vi "Autonomous.vi"   [LabVIEW 2017]
doc: "This VI starts when autonomous period begins, and will automatically be terminated when it ends. You can carry out timed or sensor driven operations directly to I/O or to subsystems without needing to return to the caller."
uses:
  Framework/Robot Global Data.vi
  <vilib>/Rock Robotics/Network Tables/NT Read String.vi
types:
  T1 = enum16{"Robot Position from the FMS", "Robot Position from the Dashboard", "Robot Position for Debug"}
  T2 = typedef "WPI_DriverStationPositionInfo.ctl" = enum16{"1", "2", "3"}
  T3 = cluster{"Auto Option":string, "Left Setpoint":dbl, "Right Setpoint":dbl, "Duration":dbl}[]
  T4 = typedef "Command Status Info.ctl" = cluster{"Name":string, "Status":T5, "notifier out":T6}
  T5 = typedef "Completion Status.ctl" = enum16{"Successful", "Aborted", "Incomplete"}
  T6 = typedef "Completion Notifier.ctl" = refnum<notifier>
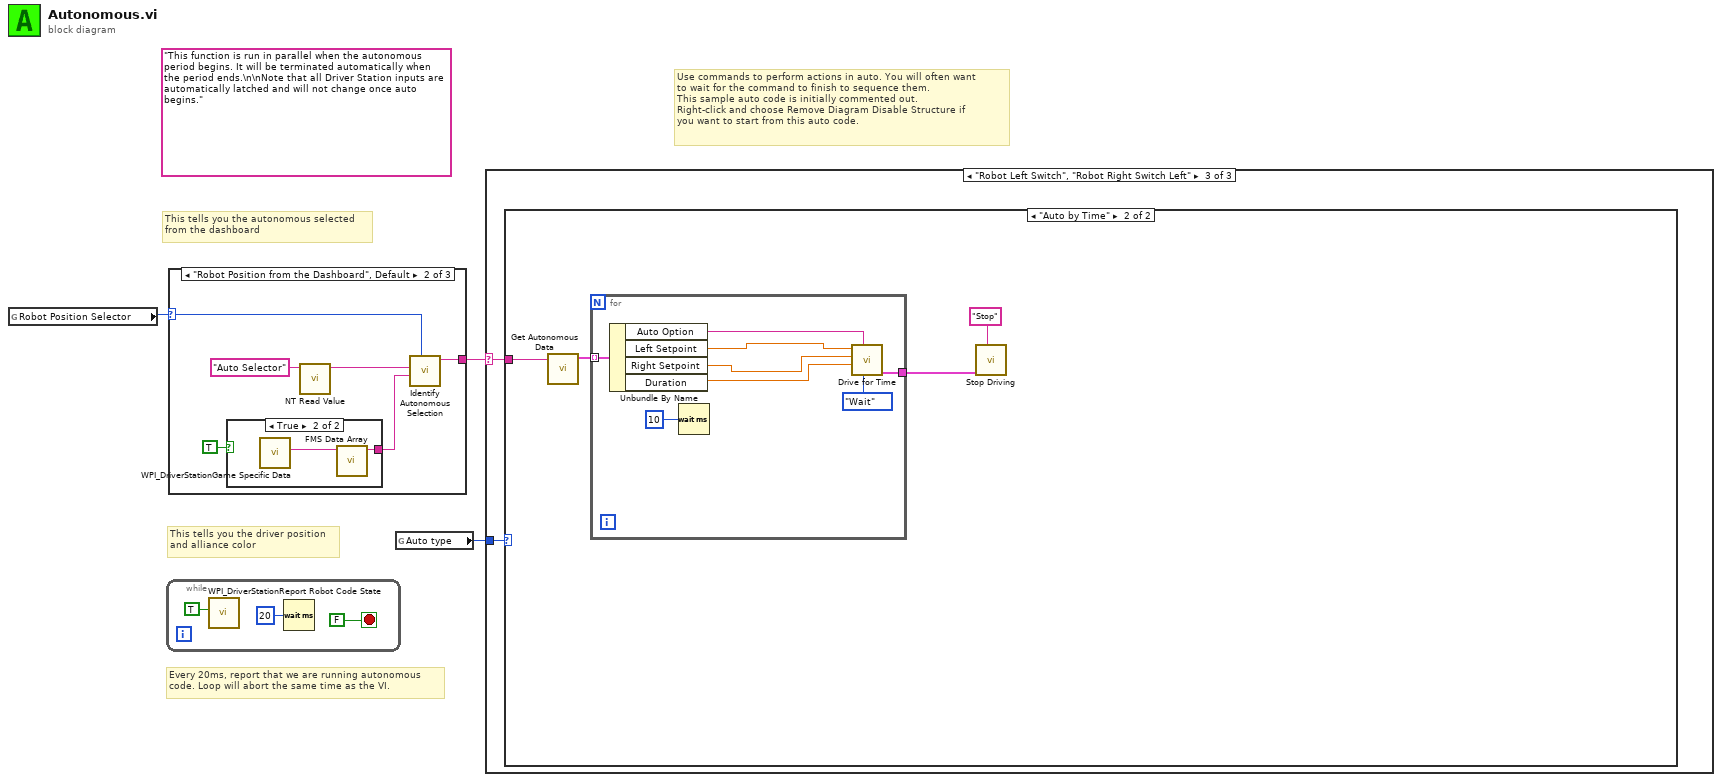
[diagram p0: block diagram]
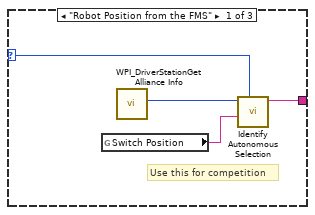
[diagram p2: hidden frame]
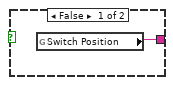
[diagram p3: hidden frame]
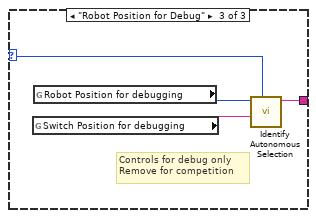
[diagram p4: hidden frame]
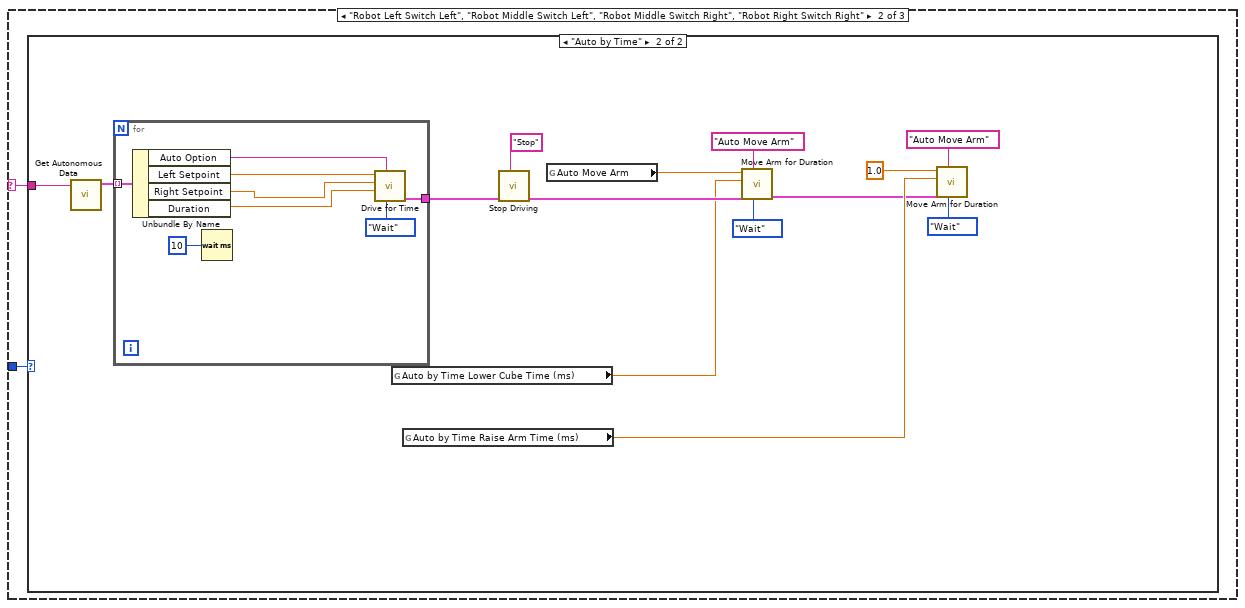
[diagram p6: hidden frame]
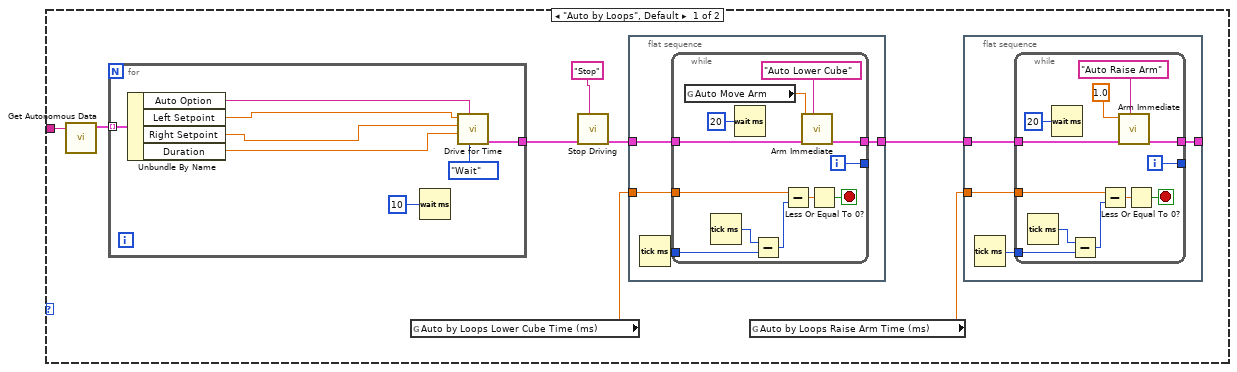
[diagram p7: hidden frame]
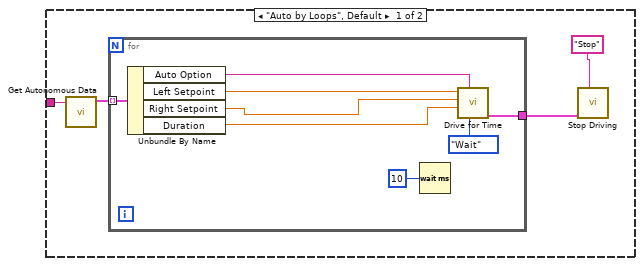
[diagram p8: hidden frame]
diagram:
  (unwired) "This function is run in parallel when the autonomous period begins. It will be terminated automatically when the period ends.\n\nNote that all Driver Station inputs are automatically latched and will not change once auto begins."
  # "This tells you the autonomous selected\nfrom the dashboard"
  # "Every 20ms, report that we are running autonomous\ncode. Loop will abort the same time as the VI."
  # "Use commands to perform actions in auto. You will often want\nto wait for the command to finish to sequence them.\nThis sample auto code is initially commented out. \nRight-click and choose Remove Diagram Disable Structure if\nyou want to start from this auto code."
  # "This tells you the driver position\nand alliance color"
  n1 = global read "Robot Global Data.vi" "Robot Position Selector"() -> (w1:T1)
  n2 = while {
    stop <- FALSE stop-if-true
    n3 = call <vilib>:"WPI_DriverStationReport Robot Code State.vi"("Autonomous"=TRUE) -> ()  [unwired: 10 in, 1 out]
    n4 = Wait (ms)(milliseconds to wait=u32 20) -> ()  [unwired: 1 out]
  }
  n5 = case shown="\"Robot Position from the Dashboard\", Default" w1 {
    selector: w1 -> [w7 w13 w20]
    tunnel: [w8 w14 w23] -> w3
    frame "Robot Position from the FMS" {
      # "Use this for competition"
      n6 = global read "Robot Global Data.vi" "Switch Position"() -> (w10:string)
      n7 = call <vilib>:"WPI_DriverStationGet Alliance Info.vi"() -> ("Position"=w9:T2)  [unwired: 11 out]
      n8 = call "Identify Autonomous Selection.vi"("Robot Position Selector"=w7, "Switch Position"=w10, "Robot Position"=w9) -> ("Autonomous Selection"=w8:string)  [unwired: 8 in]
    }
    frame "Robot Position from the Dashboard", Default {
      n9 = case shown="True" TRUE {
        tunnel: [w17 w18] -> w12
        frame False {
          n10 = global read "Robot Global Data.vi" "Switch Position"() -> (w17:string)
        }
        frame True {
          n11 = call <vilib>:"WPI_DriverStationGame Specific Data.vi"() -> ("Game Specific Data"=w19:string)  [unwired: 11 in]
          n12 = call "FMS Data Array.vi"("Game Data"=w19) -> ("Switch"=w18:string)  [unwired: 8 in, 2 out]
        }
      }
      n13 = call-poly <vilib>:"NT Read Value.vi"("Name"="Auto Selector") -> ("String"=w16:string)  [unwired: 9 in, 1 out]
      n14 = call "Identify Autonomous Selection.vi"("Robot Position Selector"=w13, "Switch Position"=w12, "Robot Position From Dashboard"=w16) -> ("Autonomous Selection"=w14:string)  [unwired: 8 in]
    }
    frame "Robot Position for Debug" {
      # "Controls for debug only\nRemove for competition"
      n15 = global read "Robot Global Data.vi" "Switch Position for debugging"() -> (w21:string)
      n16 = global read "Robot Global Data.vi" "Robot Position for debugging"() -> (w22:T2)
      n17 = call "Identify Autonomous Selection.vi"("Robot Position Selector"=w20, "Switch Position"=w21, "Robot Position"=w22) -> ("Autonomous Selection"=w23:string)  [unwired: 8 in]
    }
  }
  n18 = global read "Robot Global Data.vi" "Auto type"() -> (w2:enum16{"Auto by Time", "Auto by Loops"})
  n19 = case shown="\"Robot Left Switch\", \"Robot Right Switch Left\"" w3 {
    selector: w3 -> [_ w25 w97]
    tunnel: w2 -> [_ w24 w96]
    frame Default {
      # "You can put your main auto here, or you can right-click on the case and make any\nother frame be the default case."
      # "This is the frame that will execute if no selection is made, or if it is not recognized"
    }
    frame "Robot Left Switch Left", "Robot Middle Switch Left", "Robot Middle Switch Right", "Robot Right Switch Right" {
      n20 = case shown="\"Auto by Time\"" w24 {
        tunnel: w25 -> [w33 w87]
        frame "Auto by Loops", Default {
          n21 = call "Get Autonomous Data.vi"("Autonomous Selectin"=w33) -> ("Autonomous Data Selected"=w32:T3)  [unwired: 10 in]
          n22 = for {
            tunnel: w32 -> [w39] mode=indexing
            tunnel: [w37] -> w30
            n23 = Unbundle By Name(w39) -> ("Auto Option"=w38:string, "Left Setpoint"=w34:dbl, "Right Setpoint"=w35:dbl, "Duration"=w36:dbl)
            n24 = Wait (ms)(milliseconds to wait=u32 10 ("millisecond timer value")) -> ()  [unwired: 1 out]
            n25 = call "Drive for Time.vi"("Synchronization"=enum16{"Start", "Wait"}."Wait" ("Synchronication"), "Description"=w38, "Duration (ms)"=w36, "Right Speed"=w35, "Left Speed"=w34) -> ("Command Info Out"=w37:T4)  [unwired: 5 in, 1 out]
          }
          n26 = global read "Robot Global Data.vi" "Auto by Loops Lower Cube Time (ms)"() -> (w28:dbl)
          n27 = call "Stop Driving.vi"("Description"="Stop", "Command Info In"=w30) -> ("Command Info Out"=w29:T4)  [unwired: 9 in]
          n28 = flat-sequence {
            tunnel: [w60] -> w26
            tunnel: w29 -> [w59]
            tunnel: w28 -> [w58]
            frame #0 {
              n29 = Tick Count (ms)() -> (millisecond timer value=w61:u32)
              n30 = while {
                tunnel: w61 -> [w70]
                tunnel: w59 -> [w66]
                tunnel: [w65] -> w60
                tunnel: [w67] -> _
                tunnel: w58 -> [w63]
                i -> [w67]
                stop <- w71 stop-if-true
                n31 = global read "Robot Global Data.vi" "Auto Move Arm"() -> (w62:dbl)
                n32 = Tick Count (ms)() -> (millisecond timer value=w69:u32)
                n33 = Wait (ms)(milliseconds to wait=u32 20) -> ()  [unwired: 1 out]
                n34 = Subtract(x=w69, y=w70) -> (x-y=w73:u32)
                n35 = Subtract(x=w63, y=w73) -> (x-y=w72:dbl)
                n36 = call "Arm Immediate.vi"("Description"="Auto Lower Cube", "Command Info In"=w66, "Setpoint"=w62) -> ("Command Info Out"=w65:T4)  [unwired: 8 in]
                n37 = Less Or Equal To 0?(x=w72) -> (x <= 0?=w71:bool)
              }
            }
          }
          n38 = global read "Robot Global Data.vi" "Auto by Loops Raise Arm Time (ms)"() -> (w27:dbl)
          n39 = flat-sequence {
            tunnel: [w44] -> _
            tunnel: w26 -> [w43]
            tunnel: w27 -> [w42]
            frame #0 {
              n40 = Tick Count (ms)() -> (millisecond timer value=w45:u32)
              n41 = while {
                tunnel: w45 -> [w54]
                tunnel: w43 -> [w50]
                tunnel: [w49] -> w44
                tunnel: [w51] -> _
                tunnel: w42 -> [w46]
                i -> [w51]
                stop <- w55 stop-if-true
                n42 = Tick Count (ms)() -> (millisecond timer value=w53:u32)
                n43 = Wait (ms)(milliseconds to wait=u32 20) -> ()  [unwired: 1 out]
                n44 = Subtract(x=w53, y=w54) -> (x-y=w57:u32)
                n45 = Subtract(x=w46, y=w57) -> (x-y=w56:dbl)
                n46 = call "Arm Immediate.vi"("Description"="Auto Raise Arm", "Command Info In"=w50, "Setpoint"=1.0) -> ("Command Info Out"=w49:T4)  [unwired: 8 in]
                n47 = Less Or Equal To 0?(x=w56) -> (x <= 0?=w55:bool)
              }
            }
          }
        }
        frame "Auto by Time" {
          n48 = call "Get Autonomous Data.vi"("Autonomous Selectin"=w87) -> ("Autonomous Data Selected"=w86:T3)  [unwired: 10 in]
          n49 = for {
            tunnel: w86 -> [w93] mode=indexing
            tunnel: [w91] -> w84
            n50 = Unbundle By Name(w93) -> ("Auto Option"=w92:string, "Left Setpoint"=w88:dbl, "Right Setpoint"=w89:dbl, "Duration"=w90:dbl)
            n51 = Wait (ms)(milliseconds to wait=u32 10 ("millisecond timer value")) -> ()  [unwired: 1 out]
            n52 = call "Drive for Time.vi"("Synchronization"=enum16{"Start", "Wait"}."Wait" ("Synchronication"), "Description"=w92, "Duration (ms)"=w90, "Right Speed"=w89, "Left Speed"=w88) -> ("Command Info Out"=w91:T4)  [unwired: 5 in, 1 out]
          }
          n53 = global read "Robot Global Data.vi" "Auto by Time Lower Cube Time (ms)"() -> (w77:dbl)
          n54 = global read "Robot Global Data.vi" "Auto by Time Raise Arm Time (ms)"() -> (w76:dbl)
          n55 = call "Stop Driving.vi"("Description"="Stop", "Command Info In"=w84) -> ("Command Info Out"=w83:T4)  [unwired: 9 in]
          n56 = global read "Robot Global Data.vi" "Auto Move Arm"() -> (w74:dbl)
          n57 = call "Move Arm for Duration.vi"("Synchronization"=enum16{"Start", "Wait"}."Wait", "Description"="Auto Move Arm", "Command Info In"=w83, "Duration (ms)"=w77, "Setpoint"=w74) -> ("Command Info Out"=w75:T4)  [unwired: 6 in]
          n58 = call "Move Arm for Duration.vi"("Synchronization"=enum16{"Start", "Wait"}."Wait", "Description"="Auto Move Arm", "Command Info In"=w75, "Duration (ms)"=w76, "Setpoint"=1.0) -> ()  [unwired: 6 in, 1 out]
        }
      }
    }
    frame "Robot Left Switch", "Robot Right Switch Left" {
      n59 = case shown="\"Auto by Time\"" w96 {
        tunnel: w97 -> [w101 w113]
        frame "Auto by Loops", Default {
          n60 = call "Get Autonomous Data.vi"("Autonomous Selectin"=w101) -> ("Autonomous Data Selected"=w100:T3)  [unwired: 10 in]
          n61 = for {
            tunnel: w100 -> [w107] mode=indexing
            tunnel: [w105] -> w98
            n62 = Unbundle By Name(w107) -> ("Auto Option"=w106:string, "Left Setpoint"=w102:dbl, "Right Setpoint"=w103:dbl, "Duration"=w104:dbl)
            n63 = Wait (ms)(milliseconds to wait=u32 10 ("millisecond timer value")) -> ()  [unwired: 1 out]
            n64 = call "Drive for Time.vi"("Synchronization"=enum16{"Start", "Wait"}."Wait" ("Synchronication"), "Description"=w106, "Duration (ms)"=w104, "Right Speed"=w103, "Left Speed"=w102) -> ("Command Info Out"=w105:T4)  [unwired: 5 in, 1 out]
          }
          n65 = call "Stop Driving.vi"("Description"="Stop", "Command Info In"=w98) -> ()  [unwired: 9 in, 1 out]
        }
        frame "Auto by Time" {
          n66 = call "Get Autonomous Data.vi"("Autonomous Selectin"=w113) -> ("Autonomous Data Selected"=w112:T3)  [unwired: 10 in]
          n67 = for {
            tunnel: w112 -> [w119] mode=indexing
            tunnel: [w117] -> w110
            n68 = Unbundle By Name(w119) -> ("Auto Option"=w118:string, "Left Setpoint"=w114:dbl, "Right Setpoint"=w115:dbl, "Duration"=w116:dbl)
            n69 = Wait (ms)(milliseconds to wait=u32 10 ("millisecond timer value")) -> ()  [unwired: 1 out]
            n70 = call "Drive for Time.vi"("Synchronization"=enum16{"Start", "Wait"}."Wait" ("Synchronication"), "Description"=w118, "Duration (ms)"=w116, "Right Speed"=w115, "Left Speed"=w114) -> ("Command Info Out"=w117:T4)  [unwired: 5 in, 1 out]
          }
          n71 = call "Stop Driving.vi"("Description"="Stop", "Command Info In"=w110) -> ()  [unwired: 9 in, 1 out]
        }
      }
    }
  }
